vi "WritePosition.vi"(9 "Z":dbl, 10 "Y":dbl, 11 "X":dbl) -> ()   [LabVIEW 2017]
uses:
  Traverse-Settings-Global.vi
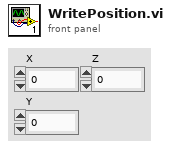
[diagram p1: front panel]
types:
  T1 = typedef "Settings-Control.ctl" = cluster{"Acceleration":dbl[], "Deceleration":dbl[], "Max Velocity":dbl[], "Speed":dbl, "Pulse/Degree":dbl, "Degre Factor":dbl[], "mm/rotation":dbl[], "Position":dbl[]}
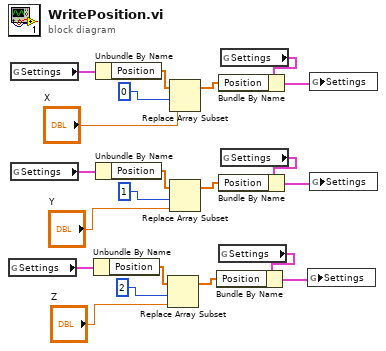
[diagram p0: block diagram]
diagram:
  n1 = global read "Traverse-Settings-Global.vi" "Settings"() -> (w6:T1)
  n2 = global read "Traverse-Settings-Global.vi" "Settings"() -> (w18:T1)
  n3 = global read "Traverse-Settings-Global.vi" "Settings"() -> (w12:T1)
  n4 = Unbundle By Name(w6) -> ("Position"=w5:dbl[])
  n5 = Unbundle By Name(w18) -> ("Position"=w17:dbl[])
  n6 = Unbundle By Name(w12) -> ("Position"=w11:dbl[])
  n7 = Replace Array Subset(array=w5, new element="Z", index=2) -> (w7:dbl[])
  n8 = Replace Array Subset(array=w17, new element="X", index=0) -> (w19:dbl[])
  n9 = Replace Array Subset(array=w11, new element="Y", index=1) -> (w13:dbl[])
  n10 = global read "Traverse-Settings-Global.vi" "Settings"() -> (w8:T1)
  n11 = Bundle By Name(cluster=w8, "Position"=w7) -> (w9:T1)
  n12 = global read "Traverse-Settings-Global.vi" "Settings"() -> (w20:T1)
  n13 = Bundle By Name(cluster=w20, "Position"=w19) -> (w21:T1)
  n14 = global read "Traverse-Settings-Global.vi" "Settings"() -> (w14:T1)
  n15 = Bundle By Name(cluster=w14, "Position"=w13) -> (w15:T1)
  n16 = global write "Traverse-Settings-Global.vi" "Settings"(w9) -> ()
  n17 = global write "Traverse-Settings-Global.vi" "Settings"(w21) -> ()
  n18 = global write "Traverse-Settings-Global.vi" "Settings"(w15) -> ()
